vi "Write Version.vi"(8 "error in (no error)":errorcluster, 10 "Build Specification Version":T1, 11 "Version Data in":refnum<class "Version Data.lvclass">) -> (0 "error out":errorcluster, 3 "Version Data out":refnum<class "Version Data.lvclass">)   [LabVIEW 2020, in "ProjectBuilder.lvlib" / "Version Data.lvclass"]
uses:
  Version Data.lvclass
  <vilib>/AppBuilder/AB_API_Simple/Build Specification Version.ctl
  <vilib>/AppBuilder/AB_API_Simple/NI_App_Builder_API.lvlib
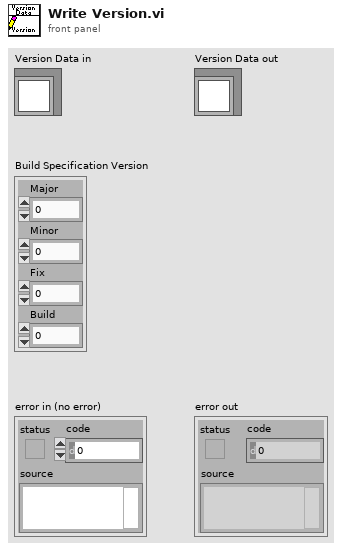
[diagram p1: front panel]
types:
  T1 = typedef "NI_App_Builder_API.lvlib/Build Specification Version.ctl" = cluster{"Major":u16, "Minor":u16, "Fix":u16, "Build":u16}
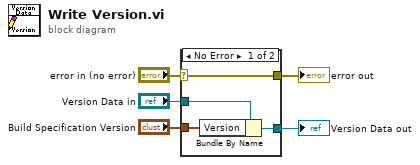
[diagram p0: block diagram]
diagram:
  n1 = case shown="No Error" "error in (no error)" {
    selector: "error in (no error)" -> [w9 w10]
    tunnel: [w9 w10] -> w4
    tunnel: [w7 w11] -> w2
    tunnel: "Version Data in" -> [w8 w11]
    tunnel: "Build Specification Version" -> [w6 _]
    frame No Error {
      n2 = Bundle By Name(cluster=w8, "Version"=w6) -> (w7:refnum<class "Version Data.lvclass">)
    }
    frame Error {
    }
  }
  "error out" <- w4
  "Version Data out" <- w2
